vi "test_CalculateSpecificationBuildOrder_SplitProjectTargetsSolution.vi"() -> (3 "Pass?":bool)   [LabVIEW 2019, in "Tests.SolutionBuilder.lvlib"]
uses:
  Tests.SolutionBuilder.lvlib
  SolutionBuilder/SolutionBuilder.lvclass
  SolutionBuilder/ProjectItem/ProjectItem.lvclass
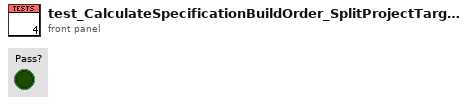
[diagram p1: front panel]
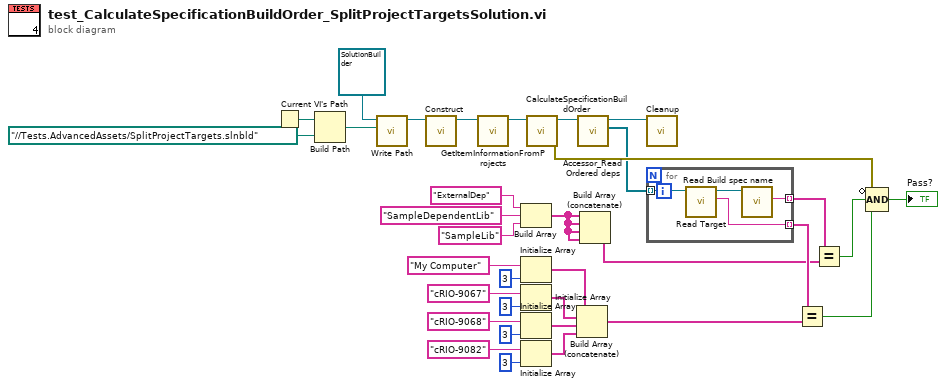
[diagram p0: block diagram]
diagram:
  n1 = Current VI's Path() -> (path=w33:path)
  n2 = Build Path(base path=w33, name or relative path=path "../../Tests.AdvancedAssets/SplitProjectTargets.slnbld" ("Path")) -> (appended path=w31:path)
  n3 = call "Write Path.vi"("Path"=w31, "SolutionBuilder in"=refnum<class "SolutionBuilder.lvclass"> refnum) -> ("SolutionBuilder out"=w30:refnum<class "SolutionBuilder.lvclass">)  [unwired: 9 in]
  n4 = call "Construct.vi"("SolutionBuilder in"=w30) -> ("SolutionBuilder out"=w28:refnum<class "SolutionBuilder.lvclass">)  [unwired: 9 in, 1 out]
  n5 = call "GetItemInformationFromProjects.vi"("SolutionBuilder in"=w28) -> ("SolutionBuilder out"=w27:refnum<class "SolutionBuilder.lvclass">)  [unwired: 9 in, 1 out]
  n6 = Build Array("ExternalDep" ("Build spec name"), "SampleDependentLib" ("Build spec name"), "SampleLib" ("Build spec name")) -> (w3:string[])
  n7 = Initialize Array("My Computer" ("Build spec name"), 3 ("dimension size")) -> (w15:string[])
  n8 = Initialize Array("cRIO-9067" ("Build spec name"), 3 ("dimension size")) -> (w14:string[])
  n9 = Initialize Array("cRIO-9068" ("Build spec name"), 3 ("dimension size")) -> (w13:string[])
  n10 = Initialize Array("cRIO-9082" ("Build spec name"), 3 ("dimension size")) -> (w8:string[])
  n11 = call "CalculateSpecificationBuildOrder.vi"("SolutionBuilder in"=w27) -> ("error out"=w24:errorcluster, "SolutionBuilder out"=w26:refnum<class "SolutionBuilder.lvclass">)  [unwired: 9 in]
  n12 = Build Array (concatenate)(w15, w14, w13, w8) -> (w7:string[])
  n13 = call "Accessor_Read Ordered deps.vi"("SolutionBuilder in"=w26) -> ("Ordered deps"=w23:refnum<class "ProjectItem.lvclass">[], "SolutionBuilder out"=w25:refnum<class "SolutionBuilder.lvclass">)  [unwired: 8 in, 1 out]
  n14 = Build Array (concatenate)(w3, w3, w3, w3) -> (w2:string[])
  n15 = call "Cleanup.vi"("SolutionBuilder in"=w25) -> ()  [unwired: 9 in, 2 out]
  n16 = for {
    tunnel: w23 -> [w37] mode=indexing
    tunnel: [w38] -> w22 mode=indexing
    tunnel: [w35] -> w12 mode=indexing
    n17 = call "Read Target.vi"("ProjectItem in"=w37) -> ("Target"=w35:string, "ProjectItem out"=w36:refnum<class "ProjectItem.lvclass">)  [unwired: 9 in]
    n18 = call "Read Build spec name.vi"("ProjectItem in"=w36) -> ("Build spec name"=w38:string)  [unwired: 9 in, 1 out]
  }
  n19 = Equal?(x=w12, y=w7) -> (x = y?=w11:bool)
  n20 = Equal?(x=w22, y=w2) -> (x = y?=w29:bool)
  n21 = Compound Arithmetic op=AND(invert w24, w29, w11) -> (→"Pass?":bool)
